vi "Led.vi"() -> ()   [LabVIEW 2014]
uses:
  <vilib>/Rock Robotics/WPI/Joystick/WPI_JoystickDevRef.ctl
  <vilib>/Rock Robotics/WPI/Joystick/WPI_JoystickDeviceEnum.ctl
panel:
  in  "JoystickDevRef":T1
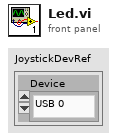
[diagram p1: front panel]
types:
  T1 = typedef "WPI_JoystickDevRef.ctl" = cluster{"Device":T2}
  T2 = typedef "WPI_JoystickDeviceEnum.ctl" = enum16{"USB 0", "USB 1", "USB 2", "USB 3", "USB 4", "USB 5"}
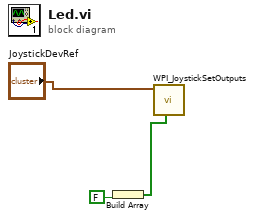
[diagram p0: block diagram]
diagram:
  n1 = Build Array(FALSE) -> (w2:bool[])
  n2 = call <vilib>:"WPI_JoystickSetOutputs.vi"("Outputs"=w2, "JoystickDevRef"="JoystickDevRef") -> ()  [unwired: 8 in, 2 out]
